vi "Relatorio.View.vi"() -> ()   [LabVIEW 2019]
uses:
  Telas.ctl
  <vilib>/Utility/miscctls.llb/LVPositionTypeDef.ctl
  <vilib>/Utility/miscctls.llb/LVPointTypeDef.ctl
  f51a7b56-5a39-448a-8df8-64775545005b.vi
  Relatorio/Relatorio_Variaveis.vi
  TelaParametrosTeste/VariaveisParametros.vi
  Relatorio/SalvarDadosTemporario.vi
panel:
  out "DadosTeste":T1
  out "ProximaTela":T2
  in  "Tab":enum32{"Page 1", "Page 2"}(tab)
  out "Graph":cluster{"X":dbl, "Y":dbl}[](graph)
  in  "TipoMedição":u16(ring) caption="Seleção forma de geração" items=["Velocidade informada"=90, "Velocidade do motor"=91]
  in  "DadosGeracao":u16(ring) caption="Dados geração:" items=["31/10.2023 20:37.11"]
  in  "Voltar":bool
  out "Info":string
  in  "Salvar":bool
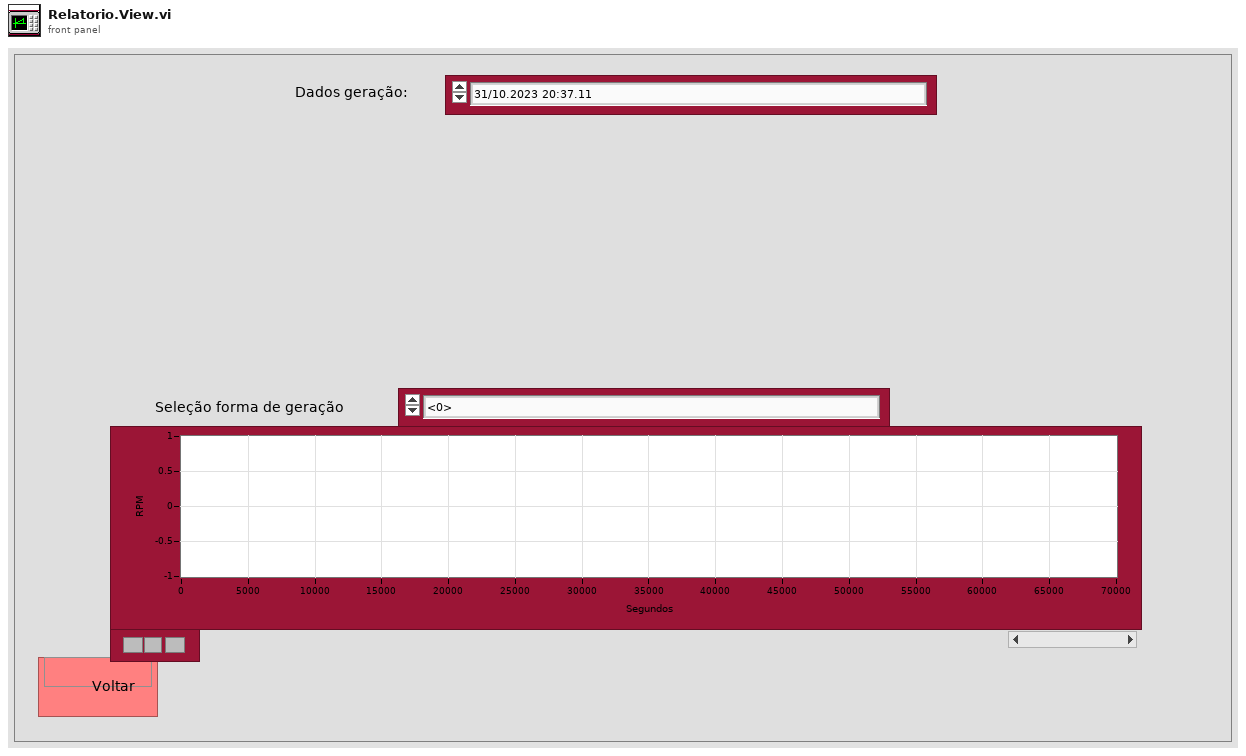
[diagram p1: front panel]
types:
  T1 = cluster{"Graph":cluster{"Descricao":string, "Graph":cluster{"X":dbl, "Y":dbl}[]}[], "Data":timestamp, "ModeloMotor":string, "ModeloInversor":string, "ModeloAeroGerador":string, "PotenciaAero":string}
  T2 = typedef "Telas.ctl" = enum16{"Selecao", "Config", "Medicao", "ParametrosTeste"}
  T3 = typedef "LVPositionTypeDef.ctl" = cluster{"Left":i32, "Top":i32}
  T4 = typedef "LVPointTypeDef.ctl" = cluster{"Horizontal":i16, "Vertical":i16}
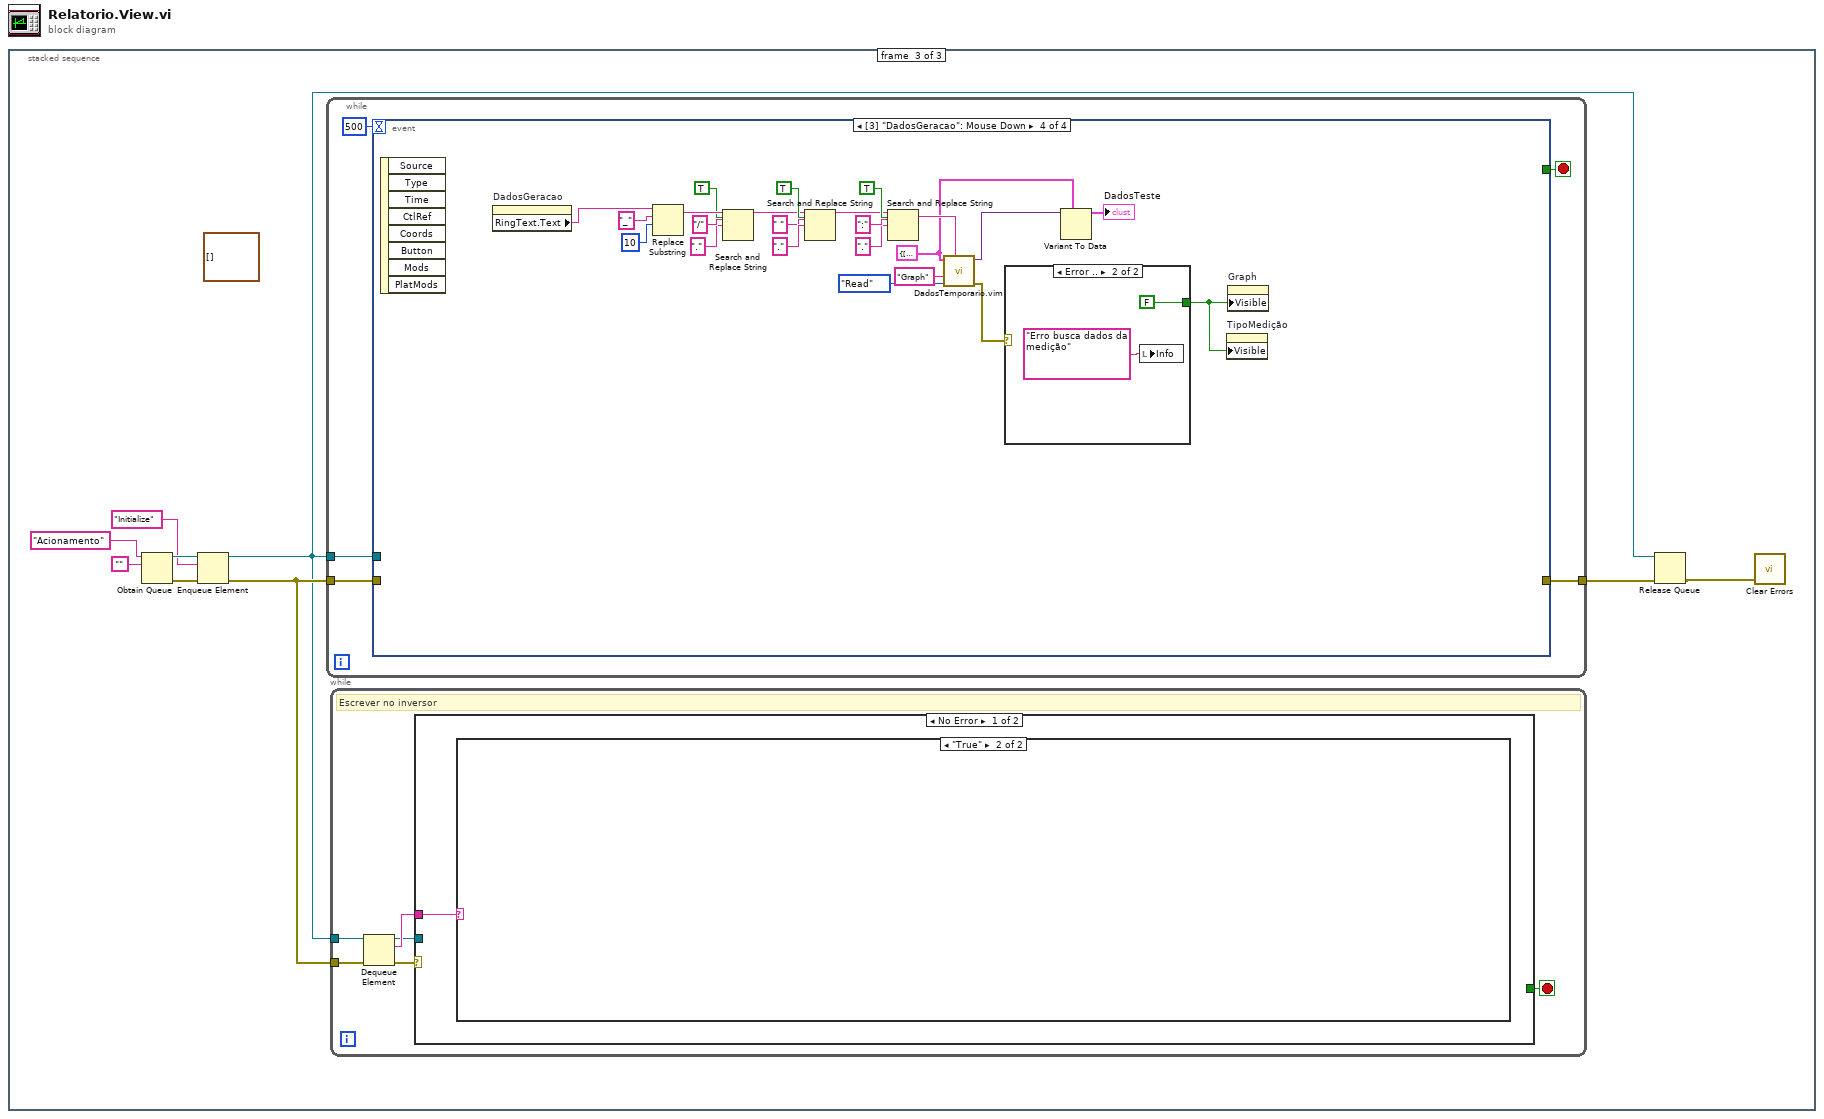
[diagram p0: block diagram]
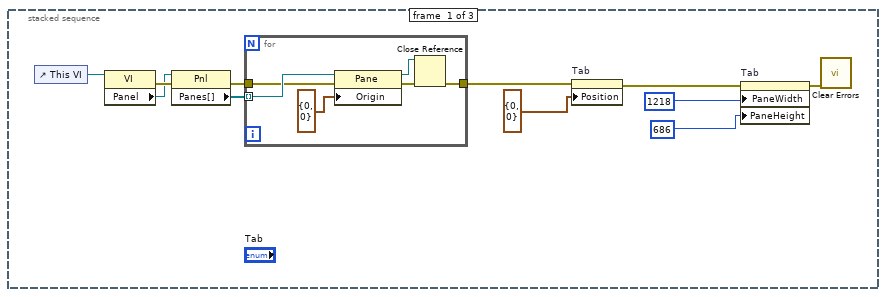
[diagram p2: hidden frame]
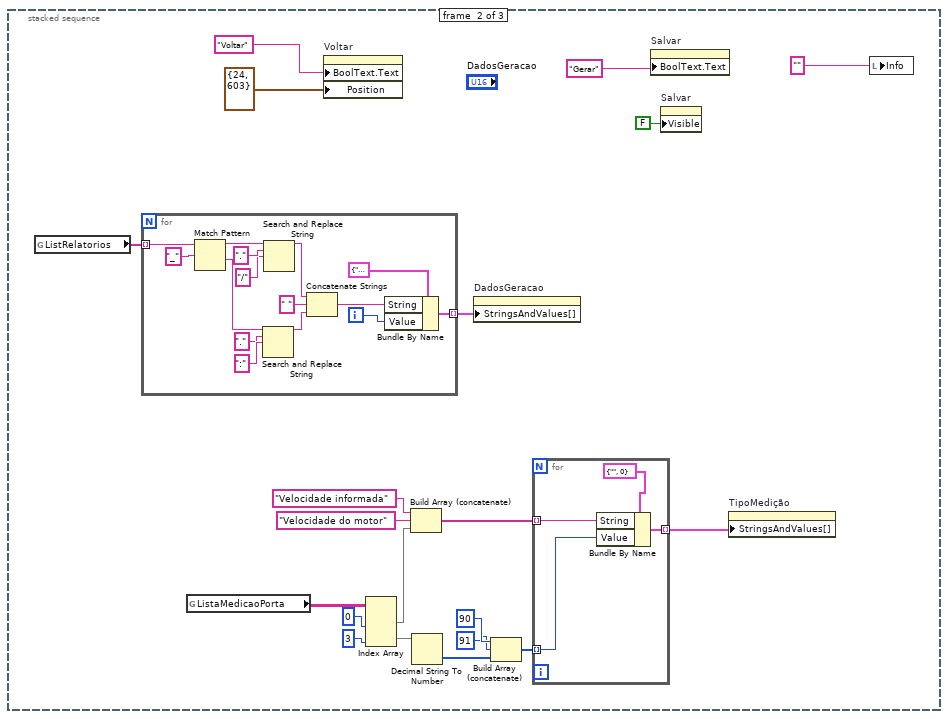
[diagram p3: hidden frame]
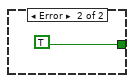
[diagram p5: hidden frame]
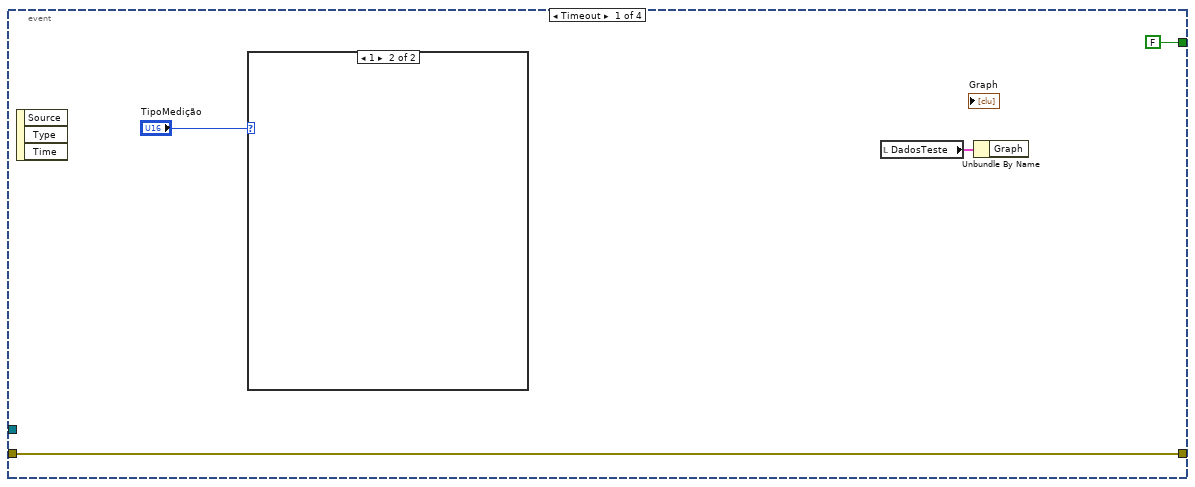
[diagram p6: hidden frame]
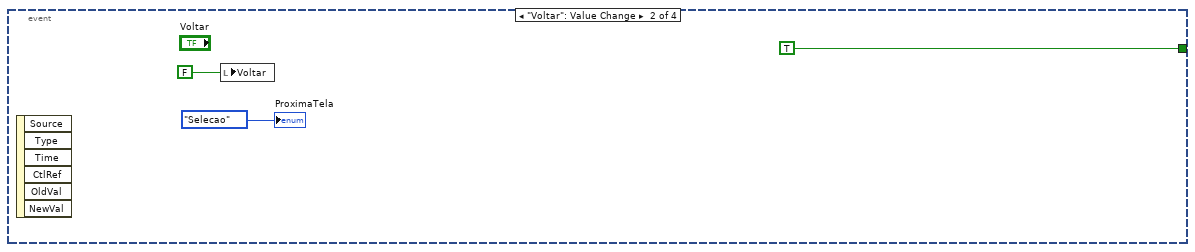
[diagram p8: hidden frame]
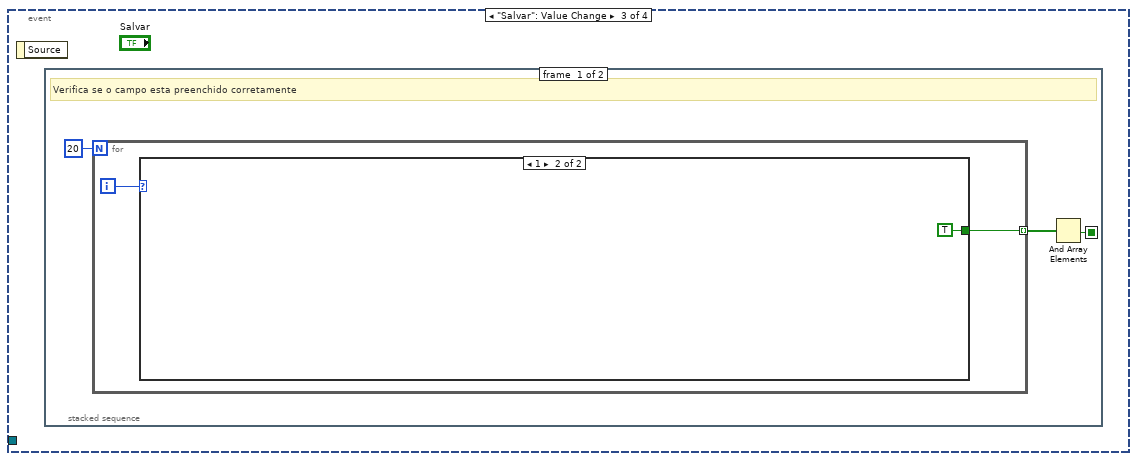
[diagram p9: hidden frame]
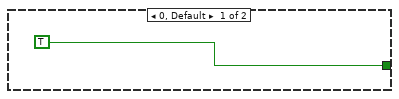
[diagram p10: hidden frame]
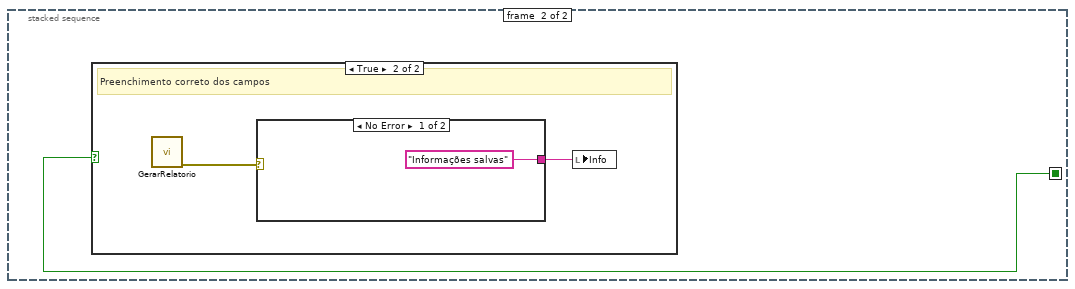
[diagram p11: hidden frame]
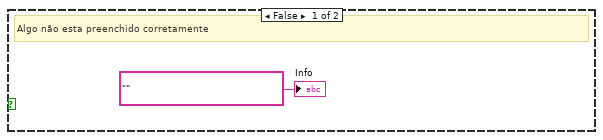
[diagram p12: hidden frame]
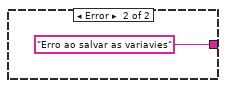
[diagram p13: hidden frame]
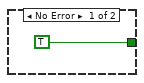
[diagram p14: hidden frame]
diagram:
  n1 = stacked-sequence {
    frame #0 {
      n2 = control-ref of="This VI"() -> (w8:refnum<vi>)
      n3 = property class="VI"(reference=w8) -> (error out=w11:errorcluster, "Panel"=w10:refnum<vi>)  [unwired: 1 in, 1 out]
      n4 = property class="Pnl"(reference=w10, error in=w11) -> (error out=w7:errorcluster, "Panes[]"=w9:refnum<vi>[])  [unwired: 1 out]
      n5 = for {
        tunnel: w9 -> [w17] mode=indexing
        tunnel: w7 -> [w13]
        tunnel: [w12] -> w6
        n6 = property class="Pane"(reference=w17, error in=w13, "Origin"=T4 {"Horizontal"=0, "Vertical"=0}) -> (reference out=w14:refnum<vi>, error out=w15:errorcluster)
        n7 = Close Reference(reference=w14, error in (no error)=w15) -> (error out=w12:errorcluster)
      }
      n8 = property on="Tab" class="TabCtl (strict)"(error in=w6, "Position"=T3 {"Left"=0, "Top"=0}) -> (error out=w5:errorcluster)  [unwired: 1 in, 1 out]
      n9 = property on="Tab" class="TabCtl (strict)"(error in=w5, "PaneWidth"=u32 1218 ("Tab Control Pane Dimension:Width"), "PaneHeight"=u32 686 ("Tab Control Pane Dimension:Height")) -> (error out=w4:errorcluster)  [unwired: 1 in, 1 out]
      n10 = call <vilib>:"Clear Errors.vi"("error in (no error)"=w4) -> ()  [unwired: 5 in, 2 out]
    }
    frame #1 {
      n11 = global read "Relatorio_Variaveis.vi" "ListRelatorios"() -> (w32:string[])
      n12 = for {
        tunnel: w32 -> [w53] mode=indexing
        tunnel: [w54] -> w31 mode=indexing
        i -> [w55]
        n13 = Match Pattern(string=w53, regular expression="_") -> (before substring=w51:string, after substring=w46:string)  [unwired: 1 in, 2 out]
        n14 = Search and Replace String(input string=w46, search string=".", replace string=":" ("replace string (\"\")")) -> (result string=w45:string)  [unwired: 5 in, 3 out]
        n15 = Search and Replace String(input string=w51, search string=".", replace string="/" ("replace string (\"\")")) -> (result string=w44:string)  [unwired: 5 in, 3 out]
        n16 = Concatenate Strings(w44, " " ("string"), w45) -> (w42:string)
        n17 = Bundle By Name(cluster=cluster{"String":string, "Value":u16} {"String"="Modo Continuo", "Value"=0}, "String"=w42, "Value"=w55) -> (w54:cluster{"String":string, "Value":u16})
      }
      n18 = global read "VariaveisParametros.vi" "ListaMedicaoPorta"() -> (w28:string[][])
      n19 = property on="Voltar" class="Bool (strict)"("BoolText.Text"="Voltar" ("Boolean Text.Text"), "Position"=T3 {"Left"=24, "Top"=603}) -> ()  [unwired: 2 in, 2 out]
      n20 = Index Array(array=w28, index (col) #1=0 ("disabled index (col)"), index (col) #2=3 ("index (col)")) -> (element #1=w29:string[], element #2=w27:string[])  [unwired: 2 in]
      n21 = Build Array (concatenate)("Velocidade informada", "Velocidade do motor", w29) -> (w30:string[])
      n22 = Decimal String To Number(string=w27) -> (number=w26:i32[])  [unwired: 2 in, 1 out]
      n23 = property on="DadosGeracao" class="Ring (strict)"("StringsAndValues[]"=w31) -> ()  [unwired: 2 in, 2 out]
      n24 = Build Array (concatenate)(90, 91, w26) -> (w25:i32[])
      n25 = for {
        tunnel: w30 -> [w41] mode=indexing
        tunnel: [w40] -> w18 mode=indexing
        tunnel: w25 -> [w39] mode=indexing
        n26 = Bundle By Name(cluster=cluster{"String":string, "Value":u16} {"String"="", "Value"=0}, "String"=w41, "Value"=w39) -> (w40:cluster{"String":string, "Value":u16})
      }
      n27 = property on="Salvar" class="Bool"("BoolText.Text"="Gerar" ("Boolean Text.Text")) -> ()  [unwired: 2 in, 2 out]
      n28 = property on="Salvar" class="Bool"("Visible"=FALSE) -> ()  [unwired: 2 in, 2 out]
      n29 = property on="TipoMedição" class="Ring (strict)"("StringsAndValues[]"=w18) -> ()  [unwired: 2 in, 2 out]
      n30 = local write "Info"("" ("InfoConfig")) -> ()
    }
    frame #2 {
      (unwired) cluster{"X":dbl, "Y":dbl}[] [] ("GraphPontos")
      n31 = Obtain Queue(name (unnamed)="Acionamento", element data type="") -> (queue out=w63:refnum<queue>, error out=w64:errorcluster)  [unwired: 3 in, 1 out]
      n32 = Enqueue Element(queue=w63, element="Initialize", error in (no error)=w64) -> (queue out=w58:refnum<queue>, error out=w59:errorcluster)  [unwired: 1 in, 1 out]
      n33 = while {
        tunnel: w58 -> [w76]
        tunnel: [w75] -> w60
        tunnel: w59 -> [w74]
        stop <- w77 stop-if-true
        n34 = event shown="[3] \"DadosGeracao\": Mouse Down" {
          selector: _ -> [_ _ _ _]
          dyn-events: _ -> [_ _ _ _]
          timeout: 500 -> [_ _ _ _]
          tunnel: [FALSE TRUE _ _] -> w77
          tunnel: w76 -> [_ _ _ _]
          tunnel: [w81 _ _ _] -> w75
          tunnel: w74 -> [w81 _ _ _]
          event Timeout {
            n35 = event-data() -> ()  [unwired: 1 in, 3 out]
            n36 = case shown="1" "TipoMedição" {
              frame 0, Default {
              }
              frame 1 {
              }
            }
            n37 = local read "DadosTeste"() -> (w79:T1)
            n38 = Unbundle By Name(w79) -> ()  [unwired: 1 out]
          }
          event "Voltar": Value Change {
            n39 = event-data() -> ()  [unwired: 1 in, 6 out]
            n40 = local write "Voltar"(FALSE ("VoltarButton")) -> ()
            "ProximaTela" <- Telas."Selecao" ("NextScreen")
          }
          event "Salvar": Value Change {
            n41 = event-data() -> ()  [unwired: 1 in, 1 out]
            n42 = stacked-sequence {
              seq-local: [w88 _] -> [_ w93]
              frame #0 {
                # "Verifica se o campo esta preenchido corretamente"
                n43 = for {
                  N: 20 -> [_]
                  tunnel: [w89] -> w87 mode=indexing
                  i -> [w90]
                  n44 = case shown="1" w90 {
                    tunnel: [TRUE TRUE] -> w89
                    frame 0, Default {
                    }
                    frame 1 {
                    }
                  }
                }
                n45 = And Array Elements(Boolean array=w87) -> (logical AND=w88:bool)
              }
              frame #1 {
                n46 = case shown="True" w93 {
                  frame False {
                    # "Algo não esta preenchido corretamente"
                    "Info" <- "" ("InfoConfig")
                  }
                  frame True {
                    # "Preenchimento correto dos campos"
                    n47 = call "GerarRelatorio.vi"() -> ("error out"=w95:errorcluster)  [unwired: 11 in]
                    n48 = case shown="No Error" w95 {
                      tunnel: ["Informações salvas" ("InfoConfig") "Erro ao salvar as variavies" ("InfoConfig")] -> w96
                      frame No Error {
                      }
                      frame Error {
                      }
                    }
                    n49 = local write "Info"(w96) -> ()
                  }
                }
              }
            }
          }
          event "DadosGeracao": Mouse Down {
            w100 = T1 {"Graph"=[], "Data"=timestamp(3705620400 s since 1904-01-01), "ModeloMotor"="", "ModeloInversor"="", "ModeloAeroGerador"="", "PotenciaAero"=""} ("Cluster")
            n50 = event-data() -> ()  [unwired: 1 in, 8 out]
            n51 = property on="DadosGeracao" class="Ring (strict)"() -> ("RingText.Text"=w107:string)  [unwired: 2 in, 2 out]
            n52 = Replace Substring(3:10 ("offset (0)"), 4:"_" ("substring (\"\")"), 5:w107) -> (1:w119:string)  [unwired: 1 in, 1 out]
            n53 = Search and Replace String(replace all?=TRUE ("replace all? (F)"), input string=w119, search string="/", replace string="." ("replace string (\"\")")) -> (result string=w109:string)  [unwired: 4 in, 3 out]
            n54 = Search and Replace String(replace all?=TRUE ("replace all? (F)"), input string=w109, search string=" ", replace string="." ("replace string (\"\")")) -> (result string=w108:string)  [unwired: 4 in, 3 out]
            n55 = Search and Replace String(replace all?=TRUE ("replace all? (F)"), input string=w108, search string=":", replace string="." ("replace string (\"\")")) -> (result string=w105:string)  [unwired: 4 in, 3 out]
            n56 = call "DadosTemporario.vim"("FileName"=w105, "Directory"="Graph", "Read/Write(Read)"=enum16{"Read", "Write"}."Read", "DataInp"=w100) -> ("ErrorOut"=w102:errorcluster, "DataOut"=w103:variant)  [unwired: 6 in]
            n57 = case shown="Error .." w102 {
              tunnel: [TRUE FALSE] -> w101
              frame No Error {
              }
              frame Error {
                n58 = local write "Info"("Erro busca dados da medição" ("Info")) -> ()
              }
            }
            n59 = Variant To Data(type=w100, Variant=w103) -> (data=→"DadosTeste":T1)  [unwired: 1 in, 1 out]
            n60 = property on="TipoMedição" class="Ring (strict)"("Visible"=w101) -> ()  [unwired: 2 in, 2 out]
            n61 = property on="Graph" class="XYGraph (strict)"("Visible"=w101) -> ()  [unwired: 2 in, 2 out]
          }
        }
      }
      n62 = while {
        tunnel: w59 -> [w70]
        tunnel: w58 -> [w69]
        stop <- w67 stop-if-true
        # "Escrever no inversor"
        n63 = Dequeue Element(queue=w69, error in (no error)=w70) -> (queue out=w66:refnum<queue>, element=w68:string, error out=w71:errorcluster)  [unwired: 1 in, 1 out]
        n64 = case shown="No Error" w71 {
          tunnel: w68 -> [w72 _]
          tunnel: [_ TRUE] -> w67
          tunnel: w66 -> [_ _]
          frame No Error {
            n65 = case shown="\"True\"" w72 {
              frame "False", Default {
              }
              frame "True" {
              }
            }
          }
          frame Error {
          }
        }
      }
      n66 = Release Queue(queue=w58, error in (no error)=w60) -> (error out=w57:errorcluster)  [unwired: 1 in, 2 out]
      n67 = call <vilib>:"Clear Errors.vi"("error in (no error)"=w57) -> ()  [unwired: 5 in, 2 out]
    }
  }
